vi "Multirecord Acquisition FPGA_20221107.vi"() -> ()   [LabVIEW 2021]
doc: "Use this VI as a template for the reconfigurable oscilloscope acquisition design. The block diagram is divided into three main loops.\n\nRegister Bus: This loop initializes the registers that are needed to support the configuration of the device. The FIFO bus, on the left, allows all the other design libraries to communicate with one another. This loop is very important to support the proper behavior of the instrument design library components.\n\nAcquisition: Acquires data from the I/O channels and writes the data into the record memory using the <B>Write</B> VI of the Multirecord Acquisition instrument design library. This VI also evaluates the various acquisition triggers and decides whether to acquire each data value in record memory. The host level VI (Fetch Record.vi) can read acquired records from the DRAM. The data is stored in 2 DRAM banks, each with 768 MB of storage.\n\nFetch: The recorded data is retrieved when the <B>Fetch Single Record</B> VI is run from the host VI. The <B>Write to Fetch DMA FIFO</B> VI writes data to the acq.fetch fifo 0 to transmit record data form the FPGA to the record fetch VIs on the host. This DMA FIFO must have a predefined name based on the instance parameter. By default, it is 0 (since the associated terminal on the <B>Create Resources DRAM Write Read</B> VI is unwired), so the connected FIFO is named acq.fetch fifo 0."
uses:
  FPGA Interface Typedefinitions/Trigger Combination Type.ctl
  Host/Clusts/AllWindowsClust.ctl
  Host/Clusts/ChannelWindowClust.ctl
  Controls/Clust/TrigSource.ctl
  Controls/Clust/WindowTriggerClust.ctl
  <instrlib>/_niInstr/Data Trigger/v1/Shared/Public/Level Configuration FXP(+-,18,1).ctl
  <instrlib>/_niInstr/Data Trigger/v1/Shared/Public/Level Configuration Trigger When.ctl
  <vilib>/Platform/TimedLoop/XDataNode/timing_clust.ctl
  <vilib>/Platform/TimedLoop/XDataNode/nitl_modes.ctl
  <vilib>/Platform/TimedLoop/XDataNode/wakeup.ctl
  Trigger/SubVIs/Types/Trigger Type.ctl
  <instrlib>/_niInstr/Data Trigger/v1/Shared/Public/Edge Configuration FXP(+-,18,1).ctl
  <instrlib>/_niInstr/Data Trigger/v1/Shared/Public/Edge Configuration Trigger Slope.ctl
  Controls/Clust/Update_Trigger_Center.ctl
  <instrlib>/_niInstr/FIFO Register Bus/v1/FPGA/niInstr FIFO Register Bus v1 FPGA.lvclass
  C:/Program Files (x86)/National Instruments/LabVIEW 2021/instr.lib/_niInstr/Instruction Framework/v1/FPGA/Interfaces/Instruction Producer/Instruction Producer.lvclass
  <instrlib>/_niInstr/Multirecord Acquisition/Common/v1/FPGA/niInstr Multirecord Acquisition Common v1 FPGA.lvclass
  C:/Program Files (x86)/National Instruments/LabVIEW 2021/instr.lib/_niInstr/Multirecord Acquisition/Interface/v1/FPGA/niInstr Multirecord Acquisition v1 FPGA.lvclass
  <vilib>/rvi/Emulation/niFpgaSctlEmulationGetInTimedLoop.vi
  <vilib>/rvi/Emulation/niFpgaEmulationReportErrorSimple.vi
  <vilib>/rvi/Emulation/niFpgaGetClockAttributes.vi
  <vilib>/rvi/Emulation/niFpgaCriticalErrorInLSC.vi
  <instrlib>/_niInstr/Multirecord Acquisition/Common/v1/FPGA/Private/Create Fetch DMA FIFO Resources U8x32.vi
  <instrlib>/_niInstr/Multirecord Acquisition/Common/v1/FPGA/Private/Create Resources DRAM U384x2 U768 Write Read.vi
  <instrlib>/_niInstr/Multirecord Acquisition/Interface/v1/FPGA/Private/Retrieve Record U16 Wrapper.vi
  <instrlib>/_niInstr/Multirecord Acquisition/Interface/v1/FPGA/Private/Write to Fetch DMA FIFO U16 Wrapper.vi
  <instrlib>/_niInstr/Basic Elements/v1/FPGA/Private/Count Up U32.vi
  <vilib>/rvi/eio/common/nirviEmuTemplateMethod_errors.vi
  <instrlib>/HSAI-RIO/Config/Group A/v1/FPGA/Digital Correction/Validate 8 Channel Data.vi
  <instrlib>/HSAI-RIO/Config/Group A/v1/FPGA/Digital Correction/Digital Correction (8 Ch).vi
  <instrlib>/HSAI-RIO/Config/Group A/v1/FPGA/Digital Correction/FIR Filter (8 Ch).vi
  DSP/SubVIs/Integer decimationx8ch.vi
  Data Type Conversion/SubVIs/Remove Overflow FXP(+-,18,1)x8ch.vi
  Trigger/Trigger FXP(+,-,18,1).vi
  Data Type Conversion/SubVIs/Data Type Conversion FXP(+-,18,1) to I16x8ch.vi
  <instrlib>/_niInstr/Channel/v1/FPGA/Private/Select and Interleave/Select And Interleave I16xNspcx8ch.vi
  <instrlib>/_niInstr/Multirecord Acquisition/Interface/v1/FPGA/Private/Write I16 Wrapper.vi
  <vilib>/Platform/TimedLoop/XDataNode/XDataNode.xnode
  <vilib>/eio/EIONode/EIONode.xnode
  <instrlib>/_niInstr/Instruction Framework/v1/FPGA/Top Level Bus/Register Configuration/Register Configuration.lvclass
  <vilib>/Platform/TimedLoop/XDataNode/XDNodeRunTimeDep.lvlib
  <instrlib>/_niInstr/Multirecord Acquisition/Interface/v1/FPGA/niInstr Multirecord Acquisition v1 FPGA.lvclass
  <vilib>/rvi/LocalResourceManager/LocalResourceManager.xnode
  <vilib>/rvi/eio/common/nirviEmuReportErrorAndStop.vi
  <vilib>/rvi/DataTransferAndStorage/Container/Common/niFpgaContainerGetUniqueNameForEmu.vi
  <vilib>/rvi/DataTransferAndStorage/Container/Common/niFpgaContainerSetEmuInfo.vi
  <instrlib>/_niInstr/Channel/v1/FPGA/niInstr Channel v1 FPGA.lvlib
  <instrlib>/_niInstr/Basic Elements/v1/FPGA/niInstr Basic Elements v1 FPGA.lvlib
  <instrlib>/HSAI-RIO/Config/Group A/v1/FPGA/Digital Correction/Digital Correction.lvclass
  <instrlib>/HSAI-RIO/Config/Group A/v1/FPGA/Config Registers/Config Registers.lvclass
  <instrlib>/_niInstr/Data Trigger/v1/Shared/niInstr Data Trigger v1 Shared.lvlib
  C:/Program Files (x86)/National Instruments/LabVIEW 2021/instr.lib/_niInstr/Multirecord Acquisition/Common/v1/FPGA/niInstr Multirecord Acquisition Common v1 FPGA.lvclass
  Emulation/SubVIs/2 Element Generate Sine Cos Data FXP(+,-,14,1).vi
  <instrlib>/_niInstr/Multirecord Acquisition/Common/v1/FPGA/Private/Create Resources DRAM U384.vi
  <instrlib>/_niInstr/Multirecord Acquisition/Common/v1/FPGA/Private/Create Resources BRAM U384.vi
  <instrlib>/_niInstr/Multirecord Acquisition/Common/v1/FPGA/Private/Create Resources BRAM U768.vi
  FPGA Interface Typedefinitions/FPGA Interface Typedefinitions.lvlib
panel:
  out "Trigger Index":u16
  out "TrigCount":u32
  out "TrigCfg 0":T1
  out "trigger Source":T4
  in  "ResetTrig":bool
  in  "UserTrig":T5
  in  "trigger.rearm delay":u16=2
  in  "start trigger":bool=TRUE
  in  "reset":bool
  in  "trigger.combination type":T7
  out "fifo reg bus data 0":u64
  out "fifo reg bus status 0":u32
  in  "fifo reg bus ctrl 0":u32
  out "overflow":bool
  in  "dsp.decimation factor":u16
  out "overload":bool
  in  "channel.enable mask":u16=65535 format="%.0b"
  in  "channel.number of channels":u8=8
  # "Register Bus Controls"
  # "FPGA"
  # "Acquisition Loop Controls"
  # "DSP"
  # "Trigger"
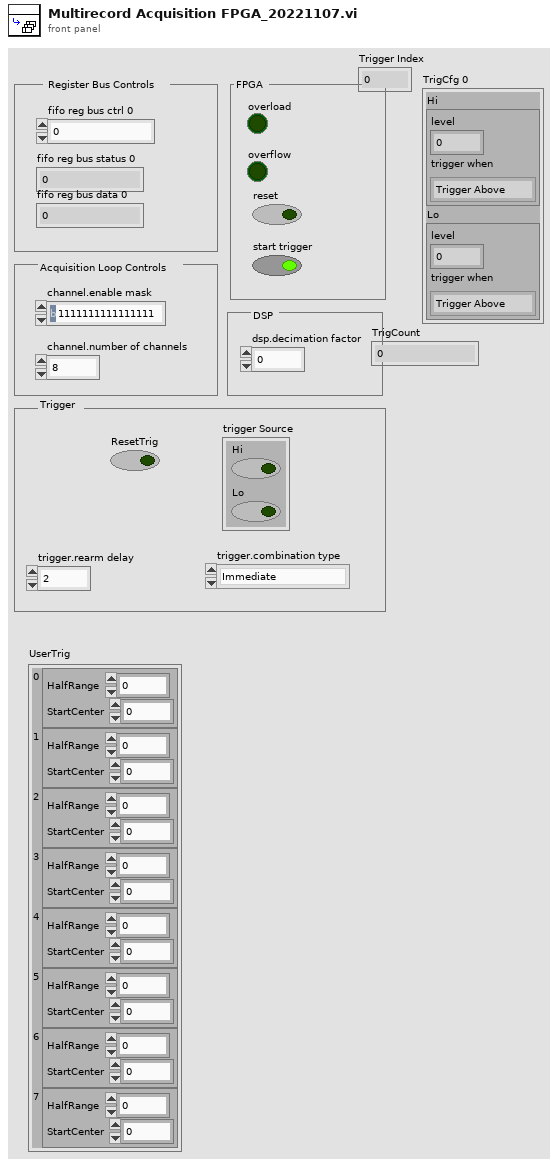
[diagram p1: front panel]
types:
  T1 = typedef "WindowTriggerClust.ctl" = cluster{"Hi":T2, "Lo":T2}
  T2 = typedef "niInstr Data Trigger v1 Shared.lvlib/Level Configuration FXP(+-,18,1).ctl" = cluster{"level":fxp<+/-,18,5>, "trigger when":T3}
  T3 = typedef "niInstr Data Trigger v1 Shared.lvlib/Level Configuration Trigger When.ctl" = enum8{"Trigger Above", "Trigger Below"}
  T4 = typedef "TrigSource.ctl" = cluster{"Hi":bool, "Lo":bool}
  T5 = typedef "AllWindowsClust.ctl" = cluster{"0":T6, "1":T6, "2":T6, "3":T6, "4":T6, "5":T6, "6":T6, "7":T6}
  T6 = typedef "ChannelWindowClust.ctl" = cluster{"HalfRange":fxp<+/-,18,5>, "StartCenter":fxp<+/-,18,5>}
  T7 = typedef "FPGA Interface Typedefinitions.lvlib/Trigger Combination Type.ctl" = enum16{"Immediate", "A", "B", "OR", "AND", "A THEN B", "B THEN A", "High Resolution"}
  T8 = cluster{"memory 1":refnum<k21>, "memory 2":refnum<k21>}
  T9 = typedef "XDNodeRunTimeDep.lvlib/timing_clust.ctl" = cluster{"Expected End [f-1]":u64, "Actual End [f-1]":u64, "Finished Late? [f-1]":bool, "Expected End [i-1]":u64, "Actual End [i-1]":u64, "Finished Late? [i-1]":bool, "Expected Start [i]":u64, "Actual Start [i]":u64, "Expected Start [f]":u64, "Actual Start [f]":u64, "Source Name":string, "Structure Name":string, "Period":i64, "Deadline":i64, "Offset":i64, "Start":i64, "Priority":i32, "Timeout":i32, "Mode":T10, "Wakeup Reason":T11, "Error":errorcluster, "Source Type":string, "Secondary Source Type":string, "Global End Time":u64, "Global Start Time":u64, "Frame Duration":u64, "Iteration Duration":u64, "Assigned CPU":i32, "I/O Scan Engine Mode":u32}
  T10 = typedef "XDNodeRunTimeDep.lvlib/nitl_modes.ctl" = enum32{"No Change", "Process missed periods, maintain original phase", "Discard missed periods, maintain original phase", "Process missed periods, ignore original phase", "Discard missed periods, ignore original phase"}
  T11 = typedef "XDNodeRunTimeDep.lvlib/wakeup.ctl" = enum32{"Normal", "Aborted", "Asynchronous wakeup", "Timing source error", "Timed loop error", "Timeout"}
  T12 = typedef "Update_Trigger_Center.ctl" = cluster{"New Center":fxp<+/-,18,5>, "apply":bool}
  T13 = typedef "Trigger Type.ctl" = enum16{"Edge", "Level", "Custom"}
  T14 = typedef "niInstr Data Trigger v1 Shared.lvlib/Edge Configuration FXP(+-,18,1).ctl" = cluster{"highLevel":fxp<+/-,18,1>, "lowLevel":fxp<+/-,18,1>, "trigger slope":T15}
  T15 = typedef "niInstr Data Trigger v1 Shared.lvlib/Edge Configuration Trigger Slope.ctl" = enum8{"Positive", "Negative"}
  T16 = cluster{"Channel 0":fxp<+/-,14,1>[], "Channel 1":fxp<+/-,14,1>[], "Channel 2":fxp<+/-,14,1>[], "Channel 3":fxp<+/-,14,1>[], "Channel 4":fxp<+/-,14,1>[], "Channel 5":fxp<+/-,14,1>[], "Channel 6":fxp<+/-,14,1>[], "Channel 7":fxp<+/-,14,1>[]}
  T17 = cluster{"Channel 0":fxp<+/-,18,1>[], "Channel 1":fxp<+/-,18,1>[], "Channel 2":fxp<+/-,18,1>[], "Channel 3":fxp<+/-,18,1>[], "Channel 4":fxp<+/-,18,1>[], "Channel 5":fxp<+/-,18,1>[], "Channel 6":fxp<+/-,18,1>[], "Channel 7":fxp<+/-,18,1>[]}
  T18 = cluster{"channel 0":fxp<+/-,18,1>[], "channel 1":fxp<+/-,18,1>[], "channel 2":fxp<+/-,18,1>[], "channel 3":fxp<+/-,18,1>[], "channel 4":fxp<+/-,18,1>[], "channel 5":fxp<+/-,18,1>[], "channel 6":fxp<+/-,18,1>[], "channel 7":fxp<+/-,18,1>[]}
  T19 = cluster{"channel 0":i16[], "channel 1":i16[], "channel 2":i16[], "channel 3":i16[], "channel 4":i16[], "channel 5":i16[], "channel 6":i16[], "channel 7":i16[]}
  T20 = typedef "niInstr Multirecord Acquisition v1 FPGA.lvclass/Timestamp.ctl" = cluster{"timestamp":u64, "valid":bool}
  T21 = typedef "niInstr Types v1 Shared.lvlib/Input Triggers.ctl" = cluster{"start":bool, "advance":bool, "reference":bool, "start trigger index":u16, "advance trigger index":u16, "reference trigger index":u16, "reference trigger correction cycle count":u32}
  T22 = typedef "niInstr Types v1 Shared.lvlib/Sample Format.ctl" = cluster{"bits per channel":u16, "samples per clock":u16, "channels":u8}
  T23 = typedef "niInstr Multirecord Acquisition v1 FPGA.lvclass/Events.ctl" = cluster{"ready for start":bool, "ready for advance":bool, "ready for reference":bool, "end of record":bool, "done":bool, "start trigger":bool, "advance trigger":bool, "reference trigger":bool, "start trigger index":u16, "advance trigger index":u16, "reference trigger index":u16}
  T24 = typedef "All_Window_Triggers_Clust.ctl" = cluster{"0":T1, "1":T1, "2":T1, "3":T1, "4":T1, "5":T1, "6":T1, "7":T1}
  T25 = typedef "niInstr Multirecord Acquisition v1 FPGA.lvclass/Retrieve Data Info.ctl" = cluster{"read request size (bits)":u64, "valid data offset (bits)":u16, "valid data size (bits)":u16, "first sample of request":bool, "last sample of request":bool, "Token":T26}
  T26 = typedef "niInstr Types v1 Shared.lvlib/Token.ctl" = cluster{"identifier":u8, "value":u32}
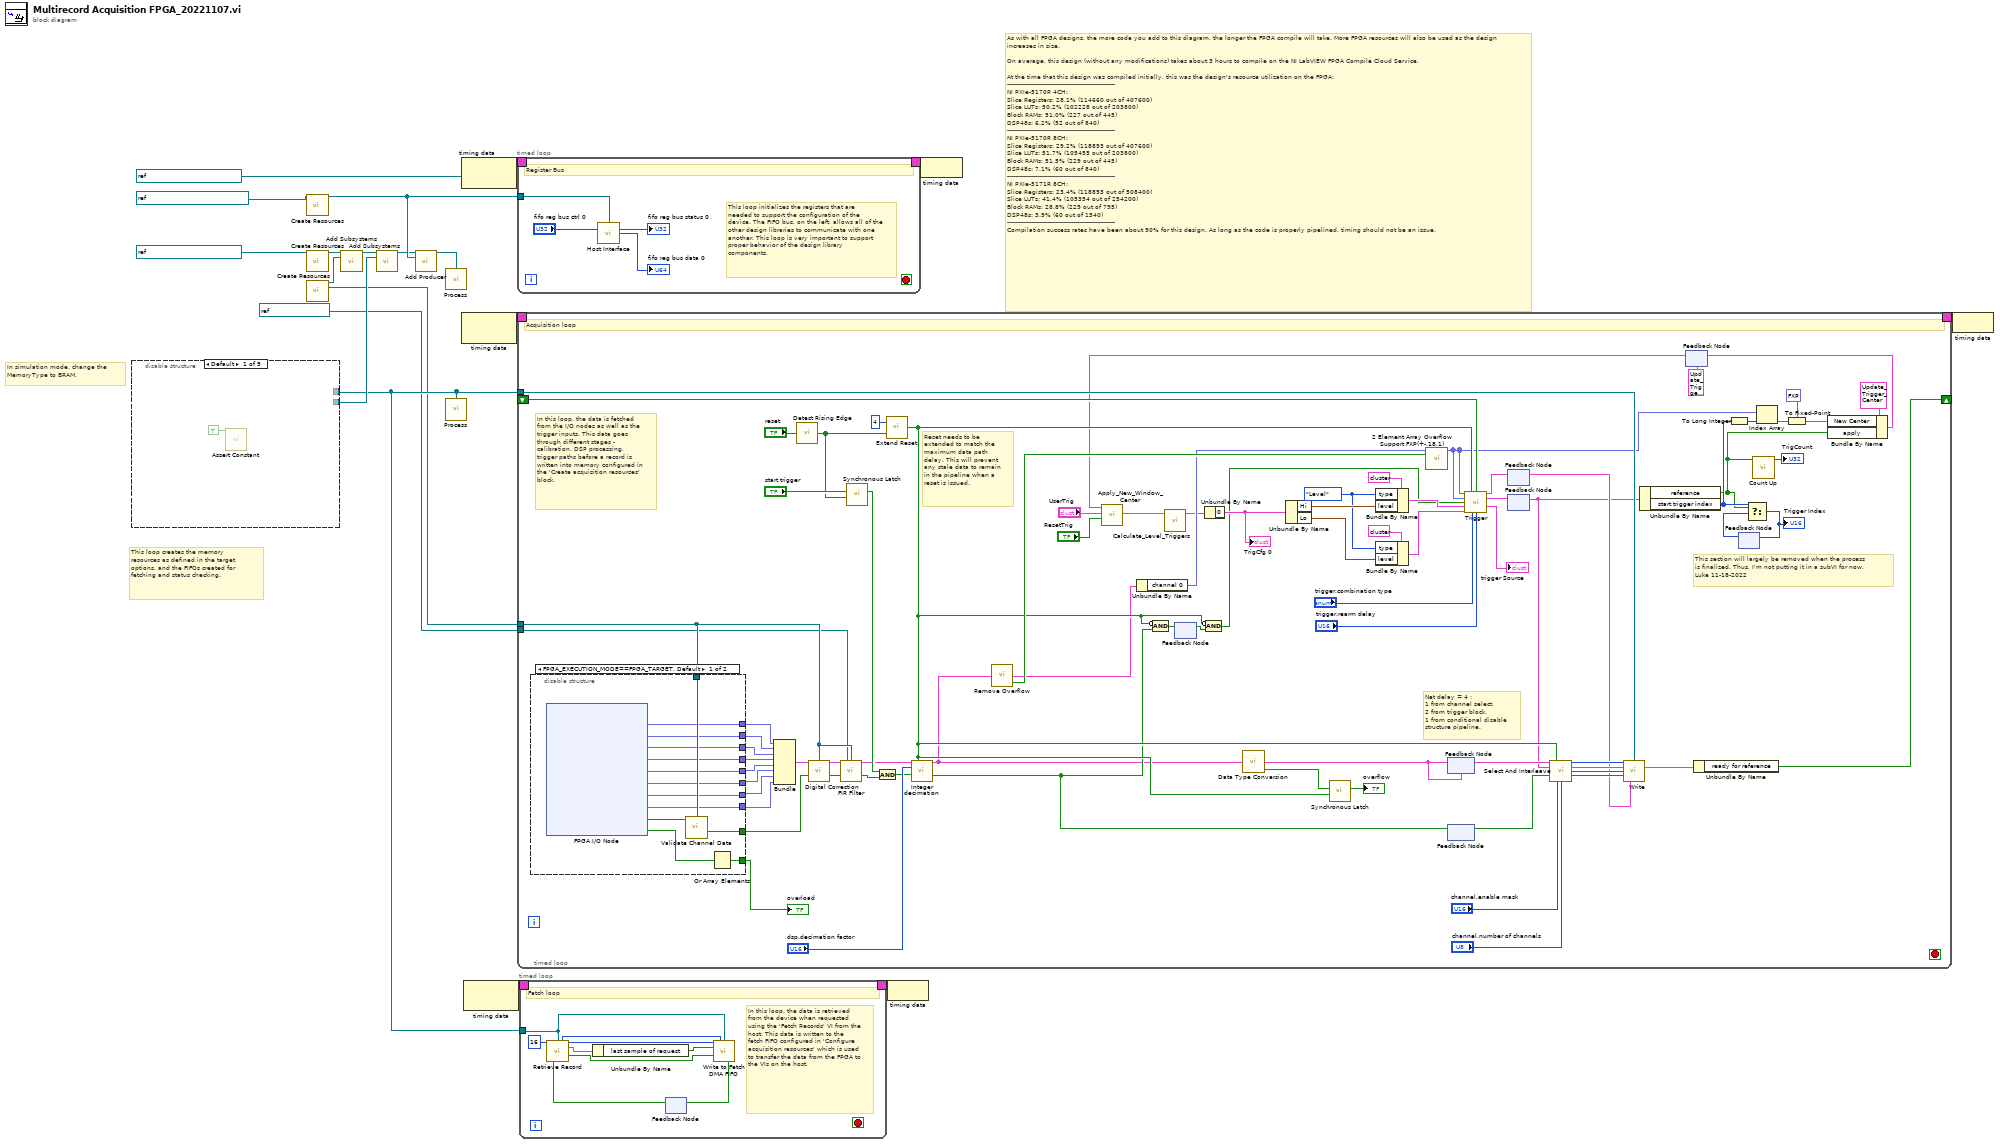
[diagram p0: block diagram]
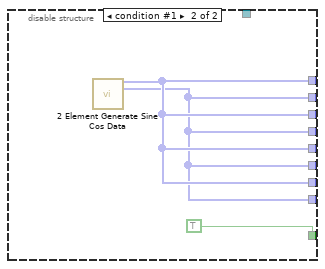
[diagram p2: hidden frame]
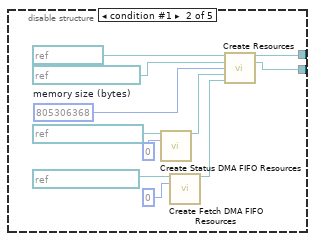
[diagram p3: hidden frame]
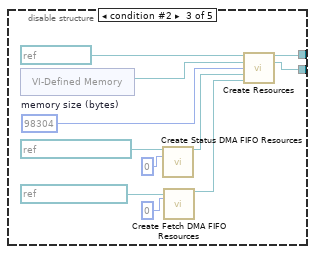
[diagram p4: hidden frame]
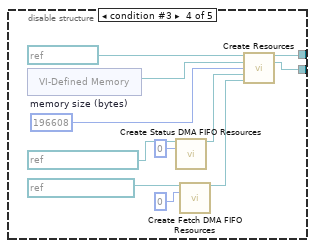
[diagram p5: hidden frame]
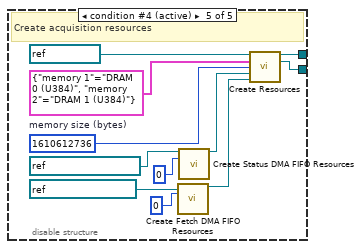
[diagram p6: hidden frame]
diagram:
  # "In simulation mode, change the MemoryType to BRAM."
  # "This loop creates the memory resources as defined in the target options, and the FIFOs created for fetching and status checking."
  # "As with all FPGA designs, the more code you add to this diagram, the longer the FPGA compile will take. More FPGA resources will also be used as the design increases in size.\n\nOn average, this design (without any modifications) takes about 3 hours to compile on the NI LabVIEW FPGA Compile Cloud Service. \n\nAt the time that this design was compiled initially, this was the design's resource utilization on the FPGA:\n------------------------------------------------------\nNI PXIe-5170R 4CH:\nSlice Registers: 28.1% (114660 out of 407600)\nSlice LUTs: 50.2% (102228 out of 203800)\nBlock RAMs: 51.0% (227 out of 445)\nDSP48s: 6.2% (52 out of 840)\n------------------------------------------------------\nNI PXIe-5170R 8CH:\nSlice Registers: 29.2% (118893 out of 407600)\nSlice LUTs: 51.7% (105455 out of 203800)\nBlock RAMs: 51.5% (229 out of 445)\nDSP48s: 7.1% (60 out of 840)\n------------------------------------------------------\nNI PXIe-5171R 8CH:\nSlice Registers: 23.4% (118893 out of 508400)\nSlice LUTs: 41.4% (105354 out of 254200)\nBlock RAMs: 28.8% (229 out of 795)\nDSP48s: 3.9% (60 out of 1540)\n------------------------------------------------------\nCompilation success rates have been about 90% for this design. As long as the code is properly pipelined, timing should not be an issue."
  n1 = disable-structure shown="Default" {
    disable-tunnel: [_ w29 w40 w51 w62] -> w4
    disable-tunnel: [_ w26 w36 w47 w59] -> w7
    frame condition #0 {
      n2 = call <instrlib>:"Assert Constant.vi"("constant terminal"=TRUE) -> ()  [unwired: 15 in]
    }
    frame condition #1 {
      w30 = u64 805306368  # memory size (bytes)
      n3 = call <instrlib>:"Create Status DMA FIFO Resources.vi"("status dma fifo in"=refnum<k21> "acq.status fifo 0" ("status dma fifo"), "fifo instance"=u8 0) -> ("status dma fifo out"=w21:refnum<class "niInstr Status FIFO v1 FPGA.lvclass">)  [unwired: 13 in]
      n4 = call-poly <instrlib>:"Create Fetch DMA FIFO Resources.vi"("fetch dma fifo in"=refnum<k21> "acq.fetch fifo 0", "fifo instance"=u8 0) -> ("fetch dma fifo out"=w27:refnum<class "niInstr Fetch FIFO v1 FPGA.lvclass">)  [unwired: 13 in]
      n5 = call-poly <instrlib>:"Create Resources.vi"("memory clock"=refnum<k21> "160MHz" ("process clock"), "memory"=refnum<k21> "DRAM 0 (U384)" ("dram"), "memory size (bytes)"=w30, "status dma fifo resources"=w21, "fetch dma fifo resources"=w27) -> ("acquisition resources"=w29:refnum<class "niInstr Multirecord Acquisition Common v1 FPGA.lvclass">, "acquisition subsystem"=w26:refnum<class "Address Space Collection.lvclass">)  [unwired: 9 in]
    }
    frame condition #2 {
      w41 = u64 98304  # memory size (bytes)
      n6 = xnode "VI-Defined Memory"() -> ("Memory Out"=w42:refnum<k21>)
      n7 = call <instrlib>:"Create Status DMA FIFO Resources.vi"("status dma fifo in"=refnum<k21> "acq.status fifo 0" ("status dma fifo"), "fifo instance"=u8 0) -> ("status dma fifo out"=w33:refnum<class "niInstr Status FIFO v1 FPGA.lvclass">)  [unwired: 13 in]
      n8 = call-poly <instrlib>:"Create Fetch DMA FIFO Resources.vi"("fetch dma fifo in"=refnum<k21> "acq.fetch fifo 0", "fifo instance"=u8 0) -> ("fetch dma fifo out"=w37:refnum<class "niInstr Fetch FIFO v1 FPGA.lvclass">)  [unwired: 13 in]
      n9 = call-poly <instrlib>:"Create Resources.vi"("memory clock"=refnum<k21> "160MHz" ("process clock"), "memory"=w42, "memory size (bytes)"=w41, "status dma fifo resources"=w33, "fetch dma fifo resources"=w37) -> ("acquisition resources"=w40:refnum<class "niInstr Multirecord Acquisition Common v1 FPGA.lvclass">, "acquisition subsystem"=w36:refnum<class "Address Space Collection.lvclass">)  [unwired: 9 in]
    }
    frame condition #3 {
      w52 = u64 196608  # memory size (bytes)
      n10 = xnode "VI-Defined Memory"() -> ("Memory Out"=w53:refnum<k21>)
      n11 = call <instrlib>:"Create Status DMA FIFO Resources.vi"("status dma fifo in"=refnum<k21> "acq.status fifo 0" ("status dma fifo"), "fifo instance"=u8 0) -> ("status dma fifo out"=w45:refnum<class "niInstr Status FIFO v1 FPGA.lvclass">)  [unwired: 13 in]
      n12 = call-poly <instrlib>:"Create Fetch DMA FIFO Resources.vi"("fetch dma fifo in"=refnum<k21> "acq.fetch fifo 0", "fifo instance"=u8 0) -> ("fetch dma fifo out"=w48:refnum<class "niInstr Fetch FIFO v1 FPGA.lvclass">)  [unwired: 13 in]
      n13 = call-poly <instrlib>:"Create Resources.vi"("memory clock"=refnum<k21> "160MHz" ("process clock"), "memory"=w53, "memory size (bytes)"=w52, "status dma fifo resources"=w45, "fetch dma fifo resources"=w48) -> ("acquisition resources"=w51:refnum<class "niInstr Multirecord Acquisition Common v1 FPGA.lvclass">, "acquisition subsystem"=w47:refnum<class "Address Space Collection.lvclass">)  [unwired: 9 in]
    }
    frame condition #4 (active) {
      w64 = u64 1610612736  # memory size (bytes)
      # "Create acquisition resources"
      n14 = call-poly <instrlib>:"Create Fetch DMA FIFO Resources.vi"("fetch dma fifo in"=refnum<k21> "acq.fetch fifo 0", "fifo instance"=u8 0) -> ("fetch dma fifo out"=w61:refnum<class "niInstr Fetch FIFO v1 FPGA.lvclass">)  [unwired: 13 in]
      n15 = call <instrlib>:"Create Status DMA FIFO Resources.vi"("status dma fifo in"=refnum<k21> "acq.status fifo 0" ("status dma fifo"), "fifo instance"=u8 0) -> ("status dma fifo out"=w56:refnum<class "niInstr Status FIFO v1 FPGA.lvclass">)  [unwired: 13 in]
      n16 = call-poly <instrlib>:"Create Resources.vi"("memory clock"=refnum<k21> "160MHz" ("process clock"), "memory"=T8 {"memory 1"="DRAM 0 (U384)", "memory 2"="DRAM 1 (U384)"}, "memory size (bytes)"=w64, "status dma fifo resources"=w56, "fetch dma fifo resources"=w61) -> ("acquisition resources"=w62:refnum<class "niInstr Multirecord Acquisition Common v1 FPGA.lvclass">, "acquisition subsystem"=w59:refnum<class "Address Space Collection.lvclass">)  [unwired: 9 in]
    }
  }
  n17 = call <instrlib>:"Create Resources.vi"("instruction fifo"=refnum<k21> "reg.host instruction fifo 0" ("FIFO")) -> ("fifo register bus"=w6:refnum<class "niInstr FIFO Register Bus v1 FPGA.lvclass">)  [unwired: 14 in]
  n18 = call <instrlib>:"Create Resources.vi"("register clock"=refnum<k21> "40 MHz Onboard Clock" ("Source Name")) -> ("register configuration"=w10:refnum<class "Register Configuration.lvclass">)  [unwired: 14 in]
  n19 = call <instrlib>:"Create Resources.vi"() -> ("config subsystems"=w8:refnum<class "Address Space Collection.lvclass">, "digital correction resources"=w1:refnum<class "Digital Correction.lvclass">)  [unwired: 14 in]
  n20 = call-dynamic "Add Subsystems.vi"("register configuration in"=w10, "subsystems"=w8) -> ("register configuration out"=w9:refnum<class "Register Configuration.lvclass">)  [unwired: 13 in]
  n21 = call-dynamic "Add Subsystems.vi"("register configuration in"=w9, "subsystems"=w7) -> ("register configuration out"=w3:refnum<class "Register Configuration.lvclass">)  [unwired: 13 in]
  n22 = call-dynamic "Add Producer.vi"("register configuration in"=w3, "instruction producer"=w6) -> ("register configuration out"=w5:refnum<class "Register Configuration.lvclass">)  [unwired: 13 in]
  n23 = call-dynamic "Process.vi"("register configuration"=w5) -> ()  [unwired: 15 in]
  n24 = call-dynamic "Process.vi"("acquisition resources"=w4) -> ()  [unwired: 15 in]
  n25 = node-c288(refnum<k21> "40 MHz Onboard Clock" ("Source Name")) -> (w19:T9)
  n26 = node-c288() -> (w17:T9)  [unwired: 1 in]
  n27 = node-c288() -> (w15:T9)  [unwired: 1 in]
  n28 = timed-loop {
    timing: w19 -> [_]
    timing-out: [_] -> w18
    tunnel: w6 -> [w68]
    stop <- _ stop-if-true
    # "This loop initializes the registers that are needed to support the configuration of the device. The FIFO bus, on the left, allows all of the other design libraries to communicate with one another. This loop is very important to support proper behavior of the design library components."
    # "Register Bus"
    n29 = call <instrlib>:"Host Interface.vi"("fifo register bus"=w68, "fifo reg bus ctrl 0"="fifo reg bus ctrl 0") -> ("fifo reg bus status 0"=→"fifo reg bus status 0":u32, "fifo reg bus data 0"=→"fifo reg bus data 0":u64)  [unwired: 12 in]
  }
  n30 = timed-loop {
    timing: w17 -> [_]
    timing-out: [_] -> w16
    tunnel: w4 -> [w150]
    tunnel: w1 -> [w127]
    shift-right: [w141] -> _
    shift-left: _ -> [w140]
    tunnel: refnum<k21> "Data Clock x2" -> [w123]
    stop <- _ stop-if-true
    w120 = Trigger_Type."Level" ("type")
    # "This section will largely be removed when the process\nis finalized. Thus, I'm not putting it in a subVI for now.\nLuke 11-18-2022"
    # "Net delay = 4 :\n1 from channel select.\n2 from trigger block.\n1 from conditional disable structure pipeline."
    # "Reset needs to be extended to match the maximum data path delay. This will prevent any stale data to remain in the pipeline when a reset is issued."
    # "In this loop, the data is fetched from the I/O nodes as well as the trigger inputs. This data goes through different stages - calibration, DSP processing, trigger paths before a record is written into memory configured in the 'Create acquisition resources' block."
    # "Acquisition loop"
    n31 = disable-structure shown="FPGA_EXECUTION_MODE==FPGA_TARGET, Default" {
      disable-tunnel: [w162 w167] -> w109
      disable-tunnel: [w161 w166] -> w108
      disable-tunnel: [w160 w167] -> w107
      disable-tunnel: [w159 w166] -> w106
      disable-tunnel: [w158 w167] -> w105
      disable-tunnel: [w157 w166] -> w104
      disable-tunnel: [w156 w167] -> w102
      disable-tunnel: [w155 w166] -> w103
      disable-tunnel: [w152 TRUE ("ADC Data Valid")] -> w100
      disable-tunnel: w127 -> [w163 _]
      disable-tunnel: [w153 _] -> w149
      frame condition #0 (active) {
        # "I/O Nodes"
        n32 = xnode "FPGA I/O Node"() -> ("Channel 0"=w162:fxp<+/-,14,1>[], "Channel 1"=w161:fxp<+/-,14,1>[], "Channel 2"=w160:fxp<+/-,14,1>[], "Channel 3"=w159:fxp<+/-,14,1>[], "Channel 4"=w158:fxp<+/-,14,1>[], "Channel 5"=w157:fxp<+/-,14,1>[], "Channel 6"=w156:fxp<+/-,14,1>[], "Channel 7"=w155:fxp<+/-,14,1>[], "Channel Data Valid"=w164:bool[], "Channel Overload"=w154:bool[])  [unwired: 10 in, 10 out]
        n33 = call-poly <instrlib>:"Validate Channel Data.vi"("channel data valid"=w164, "digital correction resources"=w163) -> ("expected data valid"=w152:bool)  [unwired: 13 in]
        n34 = Or Array Elements(Boolean array=w154) -> (logical OR=w153:bool)
      }
      frame condition #1 {
        n35 = call-poly "2 Element Generate Sine Cos Data.vi"() -> ("sine data"=w167:fxp<+/-,14,1>[], "cosine data"=w166:fxp<+/-,14,1>[])  [unwired: 14 in]
      }
    }
    "overload" <- w149
    n36 = Bundle("Channel 0"=w109, "Channel 1"=w108, "Channel 2"=w107, "Channel 3"=w106, "Channel 4"=w105, "Channel 5"=w104, "Channel 6"=w102, "Channel 7"=w103) -> (w101:T16)  [unwired: 1 in]
    n37 = call <instrlib>:"Detect Rising Edge.vi"("signal"="reset") -> ("edge detected"=w125:bool)  [unwired: 14 in]
    n38 = call-poly <instrlib>:"Digital Correction.vi"("channel data in"=w101, "digital correction resources"=w127, "input valid"=w100) -> ("corrected channel data out"=w93:T17, "output valid"=w92:bool)  [unwired: 11 in]
    n39 = call-poly <instrlib>:"FIR Filter.vi"("data in"=w93, "data clock x2"=w123, "digital correction resources"=w127, "input valid"=w92) -> ("data out"=w90:T17, "output valid"=w91:bool)  [unwired: 9 in, 1 out]
    n40 = call <instrlib>:"Synchronous Latch.vi"("clear"=w125, "set"="start trigger") -> ("out"=w131:bool)  [unwired: 9 in]
    n41 = And(x=w131, y=w91) -> (x .and. y?=w94:bool)
    n42 = call "Extend Reset.vi"("reset in"=w125, "number of cycles"=u8 4) -> ("reset out"=w114:bool)
    n43 = call-poly "Integer decimation.vi"("data in"=w90, "reset"=w114, "decimation factor"="dsp.decimation factor", "input valid"=w94) -> ("data out"=w97:T18, "output valid"=w113:bool)  [unwired: 9 in, 1 out]
    n44 = call-poly "Remove Overflow.vi"("data in"=w97) -> ("overflow"=w133:bool, "data out"=w111:T18)  [unwired: 3 in]
    n45 = Unbundle By Name(w111) -> ("channel 0"=w110:fxp<+/-,18,1>[])
    n46 = Compound Arithmetic op=AND(invert w114, w113) -> (w115:bool)
    n47 = feedback #1() -> (w116:bool)  [unwired: 1 in]
    n48 = feedback-in #1(w115) -> ()
    n49 = Compound Arithmetic op=AND(invert w114, w116) -> (w112:bool)
    n50 = call-poly "Data Type Conversion.vi"("data in"=w97) -> ("overflow"=w99:bool, "data out"=w96:T19)  [unwired: 3 in]
    n51 = call <instrlib>:"Synchronous Latch.vi"("clear"=w114, "set"=w99) -> ("out"=→"overflow":bool)  [unwired: 9 in]
    n52 = call "2 Element Array Overflow Support FXP(+-,18,1).vi"("data in"=w110, "overflow"=w133) -> ("data out"=w84:fxp<+/-,18,1>[])  [unwired: 13 in]
    n53 = feedback #2(w96) -> (w98:T19)
    n54 = feedback-in #2(w96) -> ()
    n55 = feedback #3() -> (w95:bool)  [unwired: 1 in]
    n56 = feedback-in #3(w113) -> ()
    n57 = feedback #4() -> (w117:T20)  [unwired: 1 in]
    n58 = feedback #5() -> (w88:T21)  [unwired: 1 in]
    n59 = call-poly <instrlib>:"Select And Interleave.vi"("data in"=w98, "reset"=w114, "triggers in"=w88, "input valid"=w95, "channel enable mask"="channel.enable mask", "number of channels to interleave"="channel.number of channels") -> ("interleaved data out"=w148:i16[], "triggers out"=w147:T21, "sample format out"=w146:T22, "output valid"=w145:bool)  [unwired: 5 in, 1 out]
    n60 = call-poly <instrlib>:"Write.vi"("data"=w148, "acquisition resources"=w150, "triggers"=w147, "sample format"=w146, "data valid"=w145, "timestamp"=w117) -> ("events"=w142:T23)  [unwired: 6 in, 3 out]
    n61 = Unbundle By Name(w88) -> ("reference"=w77:bool, "start trigger index"=w83:u16)
    n62 = feedback #6(T12 {"New Center"=0.0, "apply"=FALSE}) -> (w76:T12)
    n63 = call "Apply_New_Window_Center.vi"("ResetTrig"="ResetTrig", "User Trig"="UserTrig", "FeedbackTrig"=w76) -> ("AllWindows out"=w72:T5)  [unwired: 8 in]
    n64 = call "Calculate_Level_Triggers.vi"("AllWindows"=w72) -> ("All_Window_Trigs"=w73:T24)  [unwired: 8 in, 2 out]
    n65 = Unbundle By Name(w73) -> ("0"=w122:T1)
    "TrigCfg 0" <- w122
    n66 = Unbundle By Name(w122) -> ("Hi"=w121:T2, "Lo"=w119:T2)
    n67 = Bundle By Name(cluster=cluster{"type":T13, "level":T2, "edge":T14} {"type"=enum."Edge", "level"={"level"=0.0, "trigger when"=enum."Trigger Above"}, "edge"={"highLevel"=0.0, "lowLevel"=0.0, "trigger slope"=enum."Positive"}} ("trigger.A"), "type"=w120, "level"=w121) -> (w136:cluster{"type":T13, "level":T2, "edge":T14})
    n68 = Bundle By Name(cluster=cluster{"type":T13, "level":T2, "edge":T14} {"type"=enum."Edge", "level"={"level"=0.0, "trigger when"=enum."Trigger Above"}, "edge"={"highLevel"=0.0, "lowLevel"=0.0, "trigger slope"=enum."Positive"}} ("trigger.A"), "type"=w120, "level"=w119) -> (w135:cluster{"type":T13, "level":T2, "edge":T14})
    n69 = call-poly "Trigger.vi"("data A"=w84, "reset"=w114, "trigger.ready for reference"=w140, "data B"=w84, "input valid"=w112, "trigger.A"=w136, "trigger.B"=w135, "trigger.combination type"="trigger.combination type", "rearm delay"="trigger.rearm delay") -> ("timestamps"=w129:T20, "trigger.out"=w130:T21, "trigger Source"=→"trigger Source":T4)  [unwired: 3 in, 1 out]
    n70 = feedback-in #4(w129) -> ()
    n71 = feedback-in #5(w130) -> ()
    n72 = Unbundle By Name(w142) -> ("ready for reference"=w141:bool)
    n73 = To Long Integer(number=w83) -> (32bit integer=w82:i32)
    n74 = feedback #7() -> (w85:u16)  [unwired: 1 in]
    n75 = Select(t=w83, s=w77, f=w85) -> (s? t:f=w86:u16)
    "Trigger Index" <- w86
    n76 = feedback-in #7(w86) -> ()
    n77 = call-poly <instrlib>:"Count Up.vi"("increment"=w77) -> ("count out"=→"TrigCount":u32)  [unwired: 14 in]
    n78 = Index Array(array=w84, index=w82) -> (element=w81:fxp<+/-,18,1>)
    n79 = To Fixed-Point(fixed-point type=fxp<+/-,18,5> 0.0, number=w81) -> (fixed-point=w78:fxp<+/-,18,5>)
    n80 = Bundle By Name(cluster=T12 {"New Center"=0.0, "apply"=FALSE}, "New Center"=w78, "apply"=w77) -> (w75:T12)
    n81 = feedback-in #6(w75) -> ()
  }
  n82 = timed-loop {
    timing: w15 -> [_]
    timing-out: [_] -> w14
    tunnel: w4 -> [w178]
    stop <- _ stop-if-true
    # "In this loop, the data is retrieved from the device when requested using the 'Fetch Records' VI from the host. This data is written to the fetch FIFO configured in 'Configure acquisition resources' which is used to transfer the data from the FPGA to the VIs on the host."
    # "Fetch loop"
    n83 = feedback #8() -> (w176:bool)  [unwired: 1 in]
    n84 = call-poly <instrlib>:"Retrieve Record.vi"("output array size"=u16 16, "acquisition resources"=w178, "ready for output"=w176) -> ("channels"=w171:u8, "data"=w174:u16[], "retrieve data info"=w173:T25, "output valid"=w175:bool)  [unwired: 9 in]
    n85 = Unbundle By Name(w173) -> ("last sample of request"=w172:bool)
    n86 = call-poly <instrlib>:"Write to Fetch DMA FIFO.vi"("data"=w174, "channels"=w171, "acquisition resources"=w178, "last sample of request"=w172, "input valid"=w175) -> ("ready for input"=w177:bool)  [unwired: 10 in]
    n87 = feedback-in #8(w177) -> ()
  }
  n88 = node-c288(w14) -> ()
  n89 = node-c288(w18) -> ()
  n90 = node-c288(w16) -> ()
